vi "Examen01.vi"() -> ()   [LabVIEW 2020]
uses:
  <vilib>/numeric/Random Number (Range) DBL.vi
panel:
  out "Saving Data":bool
  out "rango 38 - 60?":bool
  out "numero de muestras\nmayores a maximo (60)":dbl
  out "Control ON/OFF":bool
  out "Waveform Chart":cluster{"number":dbl, dbl}(graph)
  out "valor actual sin filtrar":dbl
  in  "stop":bool
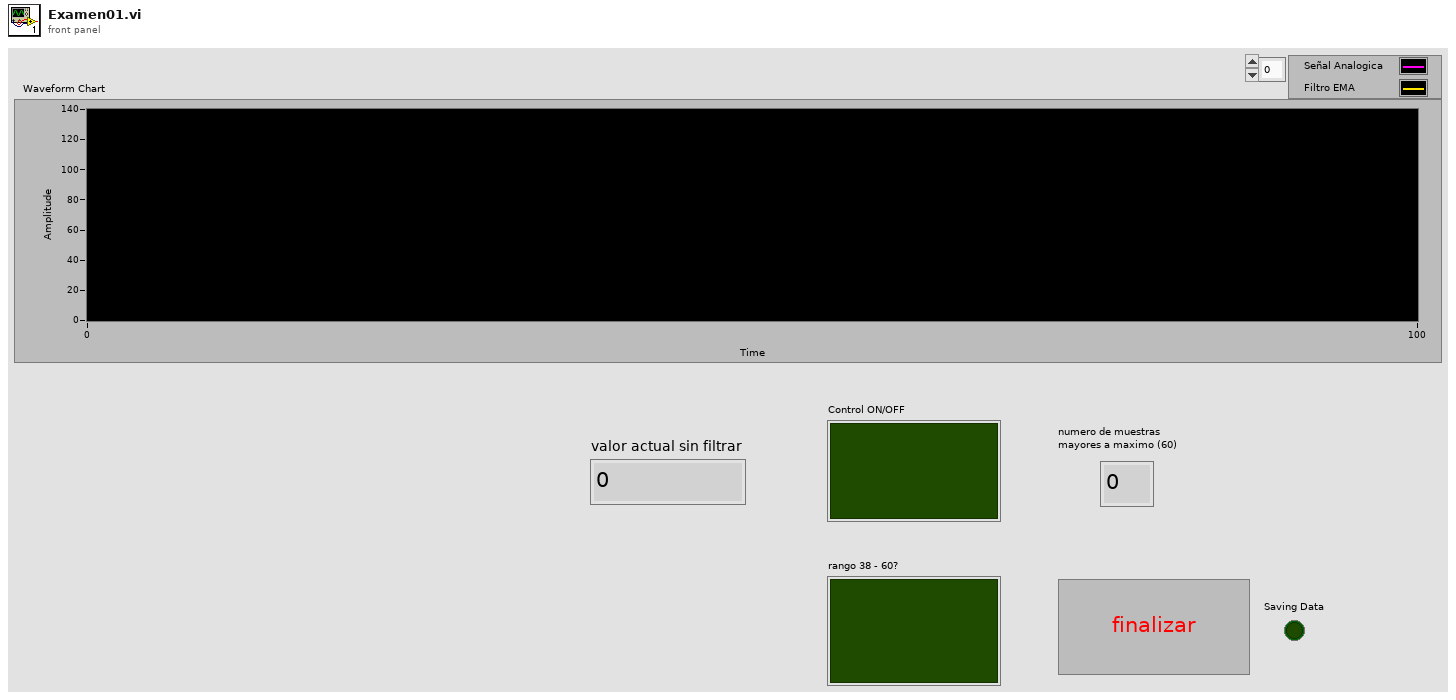
[diagram p1: front panel]
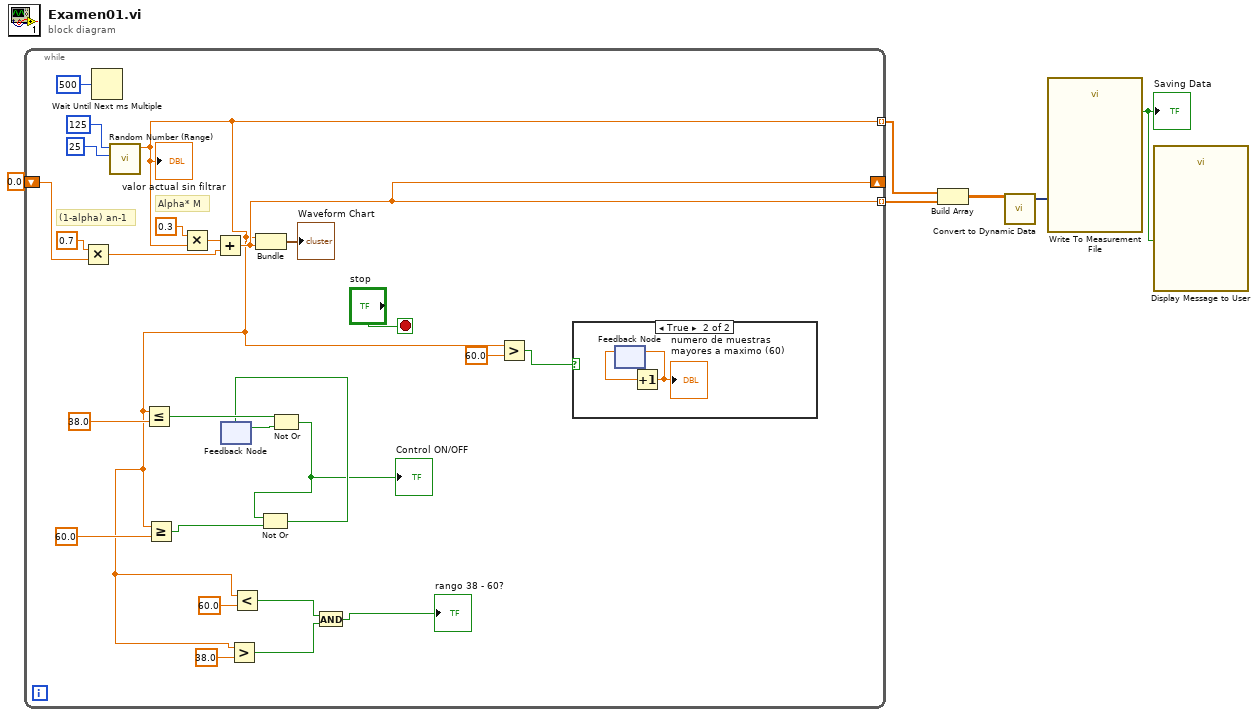
[diagram p0: block diagram]
diagram:
  n1 = while {
    shift-right: [w23] -> _
    shift-left: 0.0 -> [w28]
    tunnel: [w10] -> w5 mode=indexing
    tunnel: [w23] -> w4 mode=indexing
    stop <- "stop" stop-if-true
    # "(1-alpha) an-1"
    # "Alpha* M"
    n2 = Multiply(x=0.7, y=w28) -> (x*y=w26:dbl)
    n3 = Wait Until Next ms Multiple(millisecond multiple=u32 500) -> ()  [unwired: 1 out]
    n4 = call-poly <vilib>:"Random Number (Range).vi"("lower bound (0)"=u64 25, "upper bound (100)"=u64 125) -> ("number"=w10:dbl)  [unwired: 9 in]
    "valor actual sin filtrar" <- w10
    n5 = Less Or Equal?(x=w10, y=38.0) -> (x <= y?=w18:bool)
    n6 = Greater Or Equal?(x=w10, y=60.0) -> (x >= y?=w17:bool)
    n7 = Multiply(x=0.3, y=w10) -> (x*y=w25:dbl)
    n8 = Add(x=w25, y=w26) -> (x+y=w23:dbl)
    n9 = feedback #1() -> (w21:bool)  [unwired: 1 in]
    n10 = Greater?(x=w10, y=38.0) -> (0:w8:bool)
    n11 = Less?(x=w10, y=60.0) -> (x < y?=w9:bool)
    n12 = Bundle("number"=w10, w23) -> (→"Waveform Chart":cluster{"number":dbl, dbl})  [unwired: 1 in]
    n13 = Not Or(1:w21, 2:w18) -> (0:w15:bool)
    "Control ON/OFF" <- w15
    n14 = Not Or(1:w17, 2:w15) -> (0:w16:bool)
    n15 = feedback-in #1(w16) -> ()
    n16 = And(x=w9, y=w8) -> (x .and. y?=→"rango 38 - 60?":bool)
    n17 = Greater?(x=w10, y=60.0) -> (0:w13:bool)
    n18 = case shown="True" w13 {
      frame False {
      }
      frame True {
        n19 = feedback #2() -> (w34:dbl)  [unwired: 1 in]
        n20 = Increment(x=w34) -> (x+1=w33:dbl)
        "numero de muestras\nmayores a maximo (60)" <- w33
        n21 = feedback-in #2(w33) -> ()
      }
    }
  }
  n22 = Build Array(w5, w4) -> (w3:dbl[][])
  n23 = call "Convert to Dynamic Data"("2D Array"=w3) -> ("Dynamic Data Type"=w2:dynamicdata)  [unwired: 3 in]
  n24 = call "Write To Measurement File"("Signals"=w2) -> ("Saving Data"=w1:bool)  [unwired: 16 in, 2 out]
  "Saving Data" <- w1
  n25 = call "Display Message to User"("Enable"=w1) -> ()  [unwired: 9 in, 2 out]
